vi "XIPIN_Simulation_Reset_Generator_1_0.vi"   [LabVIEW 2017]
doc: "Simulation only Reset Generator\n------------------------------------\n<b>Need License</b> : No"
uses:
  <vilib>/rvi/XilinxIP/XIPIN_XNode/niFpgaXIPIN.xnode
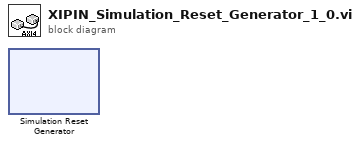
[diagram p0: block diagram]
diagram:
  n1 = xnode ("Simulation Reset Generator")() -> ()
